vi "Create New Logger (by Ref).vi"(6 "Display Format":T1, 8 "error in (no error)":errorcluster, 10 "Handlers":refnum<class "Handler.lvclass">[](array[class]), 11 "Name":string) -> (0 "error out":errorcluster)   [LabVIEW 2017, in "Error Log.lvlib" / "Logger.lvclass"]
doc: "Creates and stores a reference to a newly instantiated Logger object with the specified <b>Name</b> and <b>Handlers</b>."
uses:
  Logger.lvclass
  Handler/Handler.lvclass
  Serializer/Type Defs/Display Format.ctl
  Logger.lvclass/Logger.ctl
  Set Name.vi
  Set Display Format.vi
  Serializer/Serializer.lvlib
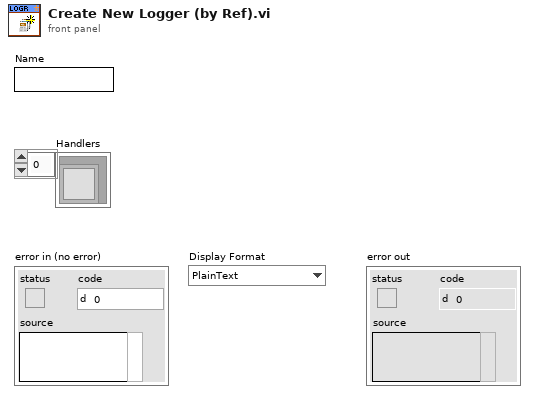
[diagram p1: front panel]
types:
  T1 = typedef "Serializer.lvlib/Display Format.ctl" = enum16{"PlainText", "PlainText.INI", "XML", "JSON"}
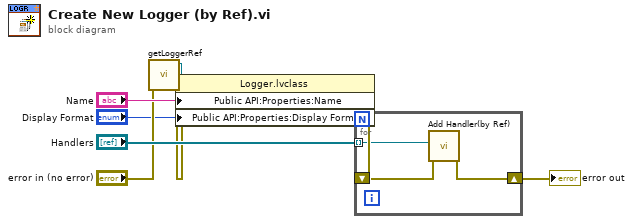
[diagram p0: block diagram]
diagram:
  n1 = call "getLoggerRef.vi"("error in (no error)"="error in (no error)") -> ("error out"=w2:errorcluster, "Logger Ref"=w6:refnum<data-value>)  [unwired: 9 in]
  n2 = property class="Logger.lvclass"(reference=w6, error in=w2, "Public API:Properties:Name"="Name", "Public API:Properties:Display Format"="Display Format") -> (error out=w7:errorcluster)  [unwired: 1 out]
  n3 = for {
    shift-right: [w10] -> w8
    shift-left: w7 -> [w11]
    tunnel: "Handlers" -> [w9] mode=indexing
    n4 = call "Add Handler(by Ref).vi"("error in (no error)"=w11, "Handler"=w9) -> ("error out"=w10:errorcluster)  [unwired: 9 in]
  }
  "error out" <- w8
